vi "Write Input Buffer.vi"(8 "error in (no error)":errorcluster, 10 "Input Buffer":sgl[](array[numeric]), 11 "ONNX Class in":refnum<class "ONNX Class.lvclass">) -> (0 "error out":errorcluster, 3 "ONNX Class out":refnum<class "ONNX Class.lvclass">)   [LabVIEW 2017, in "ONNX Class Library.lvlib" / "ONNX Class.lvclass"]
uses:
  ONNX Class.lvclass
  ONNX Class.lvclass/ONNX Class.ctl
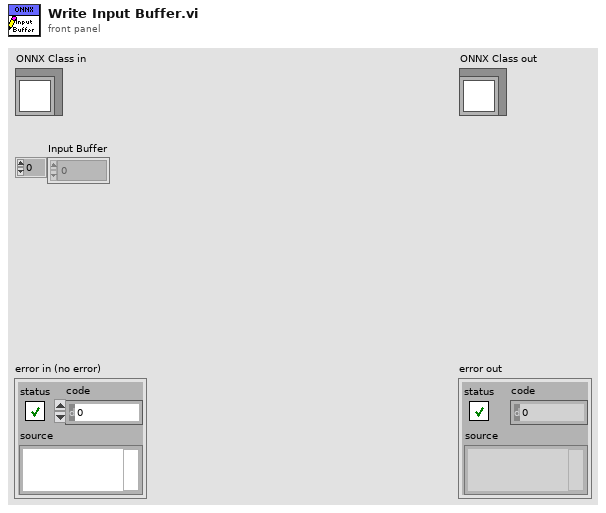
[diagram p1: front panel]
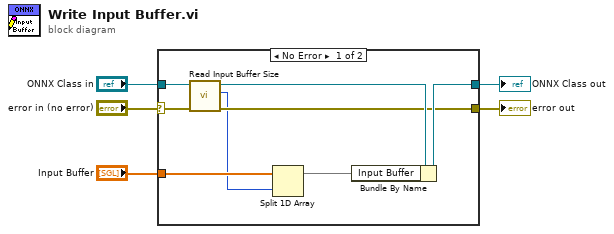
[diagram p0: block diagram]
diagram:
  n1 = case shown="No Error" "error in (no error)" {
    selector: "error in (no error)" -> [w9 w14]
    tunnel: [w8 w14] -> w4
    tunnel: [w13 w15] -> w2
    tunnel: "ONNX Class in" -> [w11 w15]
    tunnel: "Input Buffer" -> [w12 _]
    frame No Error {
      n2 = call-dynamic "Read Input Buffer Size.vi"("error in (no error)"=w9, "ONNX Class in"=w11) -> ("error out"=w8:errorcluster, "Input Buffer Size"=w6:i64, "ONNX Class out"=w10:refnum<class "ONNX Class.lvclass">)  [unwired: 7 in]
      n3 = Split 1D Array(array=w12, index=w6) -> (first subarray=w7:sgl[])  [unwired: 1 out]
      n4 = Bundle By Name(cluster=w10, "Input Buffer"=w7) -> (w13:refnum<class "ONNX Class.lvclass">)
    }
    frame Error {
    }
  }
  "error out" <- w4
  "ONNX Class out" <- w2
